vi "Configure Channel (OHM Delta).vi"(0 "VISA resource name":refnum<visa-resource-name>, 1 "Reference Channel (0001)":string="0001", 5 "Channel (0001)":string="0001", 7 "Enable Channel (True)":bool=TRUE, 9 "Type and Span":T1={"OHM Type (0 : 20ohm)"=0, "Enable Span (False)"=FALSE, "Lower Span (0.000)"=0.0, "Upper Span (20.000)"=20.0, "Bias (0)"=0.0} {"Bias (0)" format="%_6g"; "Upper Span (20.000)" min=-99999.0 max=99999.0 step=0.1 format="%.2f"; "Lower Span (0.000)" min=-99999.0 max=99999.0 step=0.1 format="%.2f"; "OHM Type (0 : 20ohm)" items=["20ohm", "200ohm", "2000ohm"]}, 11 "error in (no error)":errorcluster) -> (4 "VISA resource name out":refnum<visa-resource-name>, 6 "Channel":string, 15 "error out":errorcluster)   [LabVIEW 2020, in "Yokogawa GX Series.lvlib"]
doc: "Sets the input range as OHM (for 4 wire RTD).\n\nCommand: SRangeAI"
uses:
  <instrlib>/Yokogawa GX Series/Yokogawa GX Series.lvlib
  <instrlib>/Yokogawa GX Series/Private/OHM Range.vi
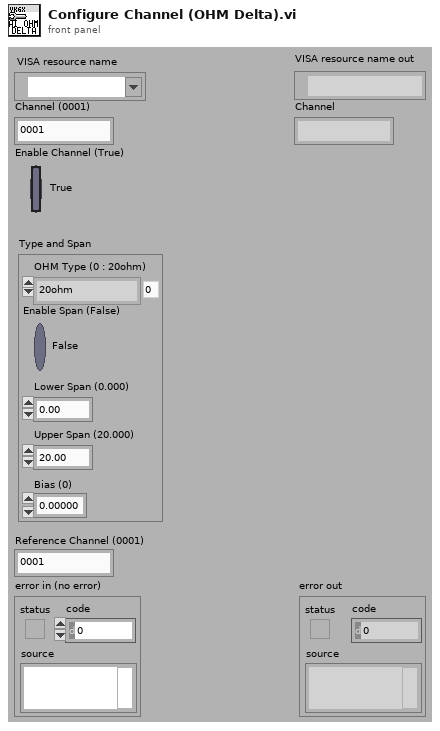
[diagram p1: front panel]
types:
  T1 = cluster{"OHM Type (0 : 20ohm)":i32, "Enable Span (False)":bool, "Lower Span (0.000)":dbl, "Upper Span (20.000)":dbl, "Bias (0)":dbl}
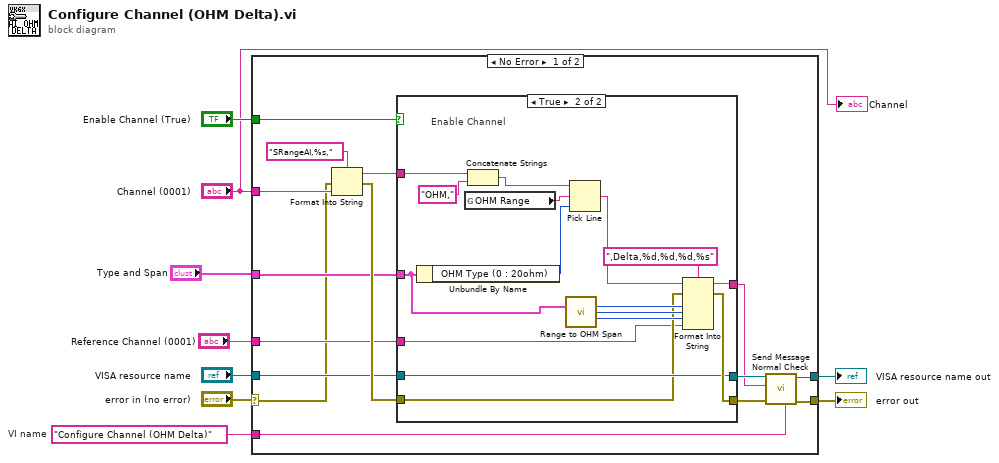
[diagram p0: block diagram]
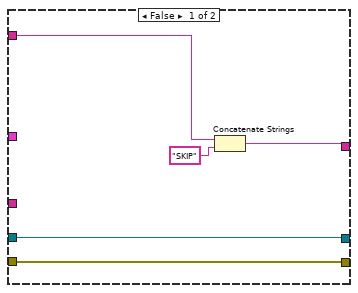
[diagram p2: hidden frame]
diagram:
  w5 = "Configure Channel (OHM Delta)"  # VI name
  n1 = case shown="No Error" "error in (no error)" {
    selector: "error in (no error)" -> [w10 w46]
    tunnel: "Enable Channel (True)" -> [w21 _]
    tunnel: "VISA resource name" -> [w20 w47]
    tunnel: "Type and Span" -> [w19 _]
    tunnel: [w15 w47] -> w7
    tunnel: [w14 w46] -> w6
    tunnel: w5 -> [w13 _]
    tunnel: "Reference Channel (0001)" -> [w12 _]
    tunnel: "Channel (0001)" -> [w11 _]
    frame No Error {
      n2 = Format Into String(format string="SRangeAI,%s,", error in=w10, w11) -> (resulting string=w22:string, error out=w23:errorcluster)  [unwired: 1 in]
      n3 = case shown="True" w21 {
        tunnel: w23 -> [w28 w32]
        tunnel: w22 -> [w29 w44]
        tunnel: [w28 w43] -> w17
        tunnel: w20 -> [w27 w33]
        tunnel: [w27 w33] -> w18
        tunnel: w19 -> [_ w40]
        tunnel: [w25 w37] -> w16
        tunnel: w12 -> [_ w31]
        frame False {
          n4 = Concatenate Strings(w29, "SKIP") -> (w25:string)
        }
        frame True {
          # "Enable Channel"
          n5 = Unbundle By Name(w40) -> ("OHM Type (0 : 20ohm)"=w39:i32)
          n6 = global read "OHM Range.vi" "OHM Range"() -> (w30:string)
          n7 = Concatenate Strings(w44, "OHM,") -> (w42:string)
          n8 = call <instrlib>:"Range to OHM Span.vi"("Range And Span"=w40) -> ("Lower Span"=w36:i32, "Upper Span"=w35:i32, "Bias"=w34:i32)  [unwired: 12 in]
          n9 = Pick Line(string ("")=w42, multi-line string=w30, line index=w39) -> (output string=w38:string)
          n10 = Format Into String(format string=",Delta,%d,%d,%d,%s", initial string=w38, error in=w32, w36, w35, w34, w31) -> (resulting string=w37:string, error out=w43:errorcluster)
        }
      }
      n11 = call <instrlib>:"Send Message Normal Check.vi"("Source (\"\")"=w13, "error in (no error)"=w17, "Send Message (\"\")"=w16, "VISA resource name"=w18) -> ("error out"=w14:errorcluster, "VISA resource name out"=w15:refnum<visa-resource-name>)  [unwired: 2 in, 4 out]
    }
    frame Error {
    }
  }
  "error out" <- w6
  "VISA resource name out" <- w7
  "Channel" <- "Channel (0001)"
